vi "Add Block Diagram Content.vi"(8 "error in (no error)":errorcluster, 10 "ModuleLoop":T1, 11 "EST Output in":refnum<class "EST Output.lvclass">) -> (0 "error out":errorcluster, 2 "Term Refnum":refnum<vi>, 3 "EST Output out":refnum<class "EST Output.lvclass">)   [LabVIEW 2025, in "EST Output.lvclass"]
uses:
  EST Output.lvclass
  VI/VI/Module.Refs.ctl
  <vilib>/Utility/miscctls.llb/LVPointTypeDef.ctl
  <vilib>/_script/New VI Object TypeDefs/NewVIObject_LVRelativePositionTypeDef.ctl
  <vilib>/_script/New VI Object TypeDefs/NewVIObject_LVRelativeDirectionTypeDef.ctl
  <vilib>/Utility/miscctls.llb/LVPoint32TypeDef.ctl
  EST Output.lvclass/EST Output.ctl
  Signal/Read IP Core Path.vi
  Signal/Read Signal Name.vi
  VI/Structures/Structures.lvclass
  Signal/Signal.lvclass
  VI/VI/VI.lvclass
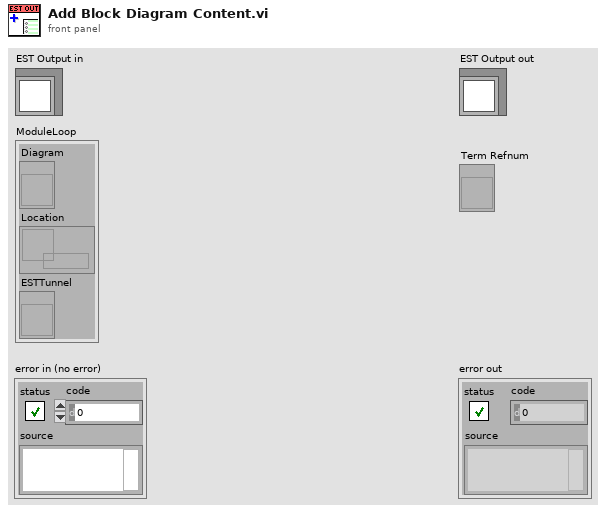
[diagram p1: front panel]
types:
  T1 = typedef "VI.lvclass/Module.Refs.ctl" = cluster{"Diagram":refnum<vi>, "Location":refnum<data-value>, "ESTTunnel":refnum<vi>}
  T2 = typedef "NewVIObject_LVRelativePositionTypeDef.ctl" = cluster{"Refnum":refnum<vi>, "Relative Direction":T3, "Point32":T4}
  T3 = typedef "NewVIObject_LVRelativeDirectionTypeDef.ctl" = enum32{"Right", "Left", "Top", "Bottom", "Top Right", "Top Left", "Bottom Right", "Bottom Left"}
  T4 = typedef "LVPoint32TypeDef.ctl" = cluster{"Horizontal":i32, "Vertical":i32}
  T5 = typedef "LVPointTypeDef.ctl" = cluster{"Horizontal":i16, "Vertical":i16}
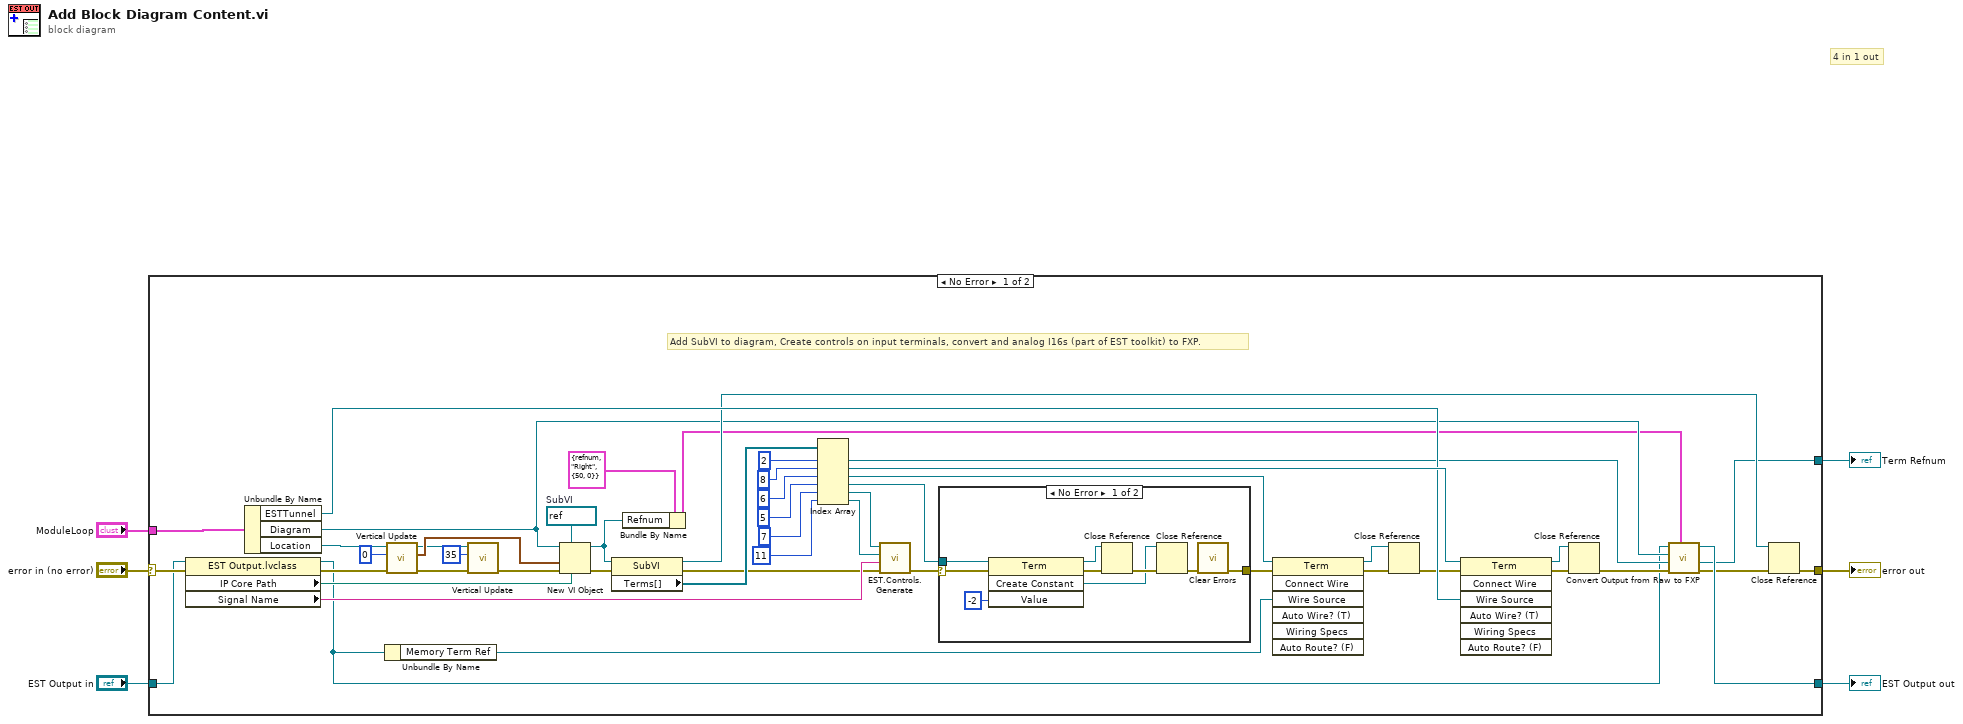
[diagram p0: block diagram]
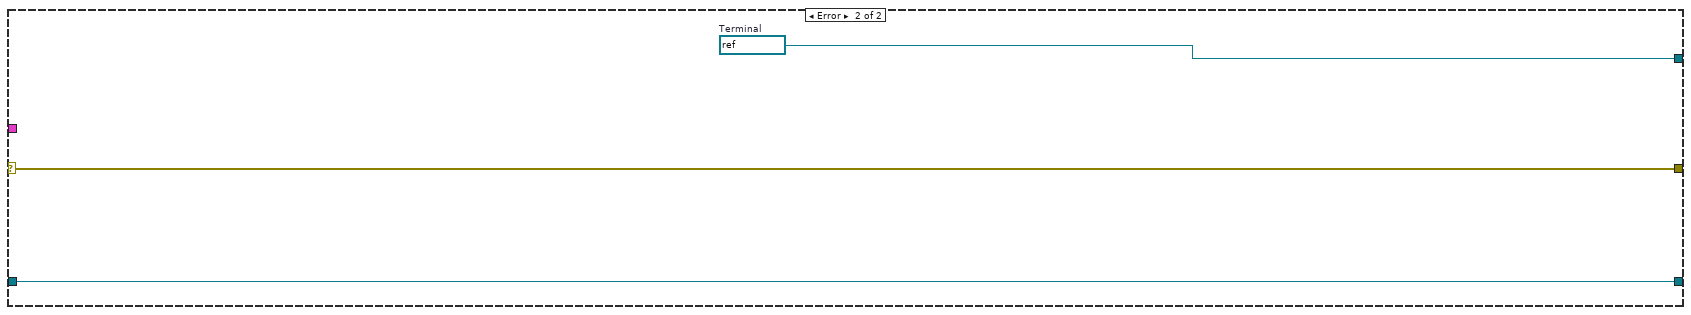
[diagram p3: hidden frame]
diagram:
  # "4 in 1 out"
  n1 = case shown="No Error" "error in (no error)" {
    selector: "error in (no error)" -> [w16 w68]
    tunnel: "ModuleLoop" -> [w55 _]
    tunnel: [w18 w68] -> w5
    tunnel: [w7 w66] -> w4
    tunnel: "EST Output in" -> [w15 w67]
    tunnel: [w9 w67] -> w2
    frame No Error {
      w51 = refnum<vi> refnum  # SubVI
      # "Add SubVI to diagram, Create controls on input terminals, convert and analog I16s (part of EST toolkit) to FXP."
      n2 = property class="EST Output.lvclass"(reference=w15, error in=w16) -> (reference out=w10:refnum<class "EST Output.lvclass">, error out=w32:errorcluster, "IP Core Path"=w37:path, "Signal Name"=w38:string)
      n3 = Unbundle By Name(w55) -> ("ESTTunnel"=w27:refnum<vi>, "Diagram"=w12:refnum<vi>, "Location"=w34:refnum<data-value>)
      n4 = Unbundle By Name(w10) -> ("Memory Term Ref"=w36:refnum<vi>)
      n5 = call "Vertical Update.vi"("error in (no error)"=w32, "Vertical Change"=i16 0, "Location"=w34) -> ("error out"=w29:errorcluster, "location out"=w33:T5, "Location"=w30:refnum<data-value>)  [unwired: 6 in]
      n6 = call "Vertical Update.vi"("error in (no error)"=w29, "Vertical Change"=i16 35, "Location"=w30) -> ("error out"=w28:errorcluster)  [unwired: 6 in, 2 out]
      n7 = New VI Object(vi object class=w51, owner refnum=w12, position/next to=w33, 6:w37, 8:w28) -> (object refnum=w19:refnum<vi>, 0:w54:errorcluster)  [unwired: 3 in]
      n8 = property class="SubVI"(reference=w19, error in=w54) -> (reference out=w17:refnum<vi>, error out=w20:errorcluster, "Terms[]"=w52:refnum<vi>[])
      n9 = Bundle By Name(cluster=T2 {"Refnum"=refnum, "Relative Direction"=enum."Right", "Point32"={"Horizontal"=50, "Vertical"=0}} ("Relative Position"), "Refnum"=w19) -> (w11:T2)
      n10 = Index Array(array=w52, index #1=2 ("index"), index #2=8 ("index"), index #3=6 ("index"), index #4=5 ("index"), index #5=7 ("index"), index #6=11 ("index")) -> (element #1=w13:refnum<vi>, element #2=w42:refnum<vi>, element #3=w45:refnum<vi>, element #4=w47:refnum<vi>, element #5=w40:refnum<vi>, element #6=w41:refnum<vi>)
      n11 = call "EST.Controls.Generate.vi"("error in (no error)"=w20, "Signal"=w38, "Input.Ref"=w41, "Settings.Ref"=w40) -> ("error out"=w39:errorcluster)  [unwired: 7 in]
      n12 = case shown="No Error" w39 {
        selector: w39 -> [w62 w65]
        tunnel: w47 -> [w64 _]
        tunnel: [w59 w65] -> w46
        frame No Error {
          n13 = invoke class="Term" method="Create Constant"(reference=w64, error in=w62, "Value"=i8 -2 ("shift")) -> (reference out=w60:refnum<vi>, error out=w61:errorcluster, "Create Constant"=w56:refnum<vi>)  [unwired: 1 in, 1 out]
          n14 = Close Reference(reference=w60, error in (no error)=w61) -> (error out=w58:errorcluster)
          n15 = Close Reference(reference=w56, error in (no error)=w58) -> (error out=w57:errorcluster)
          n16 = call <vilib>:"Clear Errors.vi"("error in (no error)"=w57) -> ("error out"=w59:errorcluster)  [unwired: 5 in, 1 out]
        }
        frame Error {
        }
      }
      n17 = invoke class="Term" method="Connect Wire"(reference=w45, error in=w46, "Wire Source"=w36) -> (reference out=w24:refnum<vi>, error out=w23:errorcluster)  [unwired: 4 in, 5 out]
      n18 = Close Reference(reference=w24, error in (no error)=w23) -> (error out=w22:errorcluster)
      n19 = invoke class="Term" method="Connect Wire"(reference=w42, error in=w22, "Wire Source"=w27) -> (reference out=w26:refnum<vi>, error out=w25:errorcluster)  [unwired: 4 in, 5 out]
      n20 = Close Reference(reference=w26, error in (no error)=w25) -> (error out=w14:errorcluster)
      n21 = call "Convert Output from Raw to FXP.vi"("Relative Position"=w11, "error in (no error)"=w14, "Term Refnum"=w13, "Diagram"=w12, "Signal in"=w10) -> ("error out"=w8:errorcluster, "Term Refnum out"=w7:refnum<vi>, "Signal out"=w9:refnum<class "EST Output.lvclass">)  [unwired: 4 in]
      n22 = Close Reference(reference=w17, error in (no error)=w8) -> (error out=w18:errorcluster)
    }
    frame Error {
      w66 = refnum<vi> refnum  # Terminal
    }
  }
  "error out" <- w5
  "EST Output out" <- w2
  "Term Refnum" <- w4
